vi "Configure Device.vi"(8 "error in":errorcluster, 11 "Alicat Device in":refnum<class "Alicat Device.lvclass">) -> (0 "error out":errorcluster, 3 "Alicat Device out":refnum<class "Alicat Device.lvclass">)   [LabVIEW 2015, in "Alicat Device.lvclass"]
uses:
  Alicat Device.lvclass
  Configurable Device/Configurable Device.lvclass/Configurable Device.ctl
  Reusable/Session APIs/File Access/Config Data/Config Data.lvclass/Config Data.ctl
  Alicat Device.lvclass/Alicat Device.ctl
  Configurable Device/Read Handle.vi
  <vilib>/Utility/config.llb/Read Key (String).vi
  <vilib>/Utility/config.llb/Read Key (Double).vi
  <vilib>/Utility/config.llb/Read Key (Boolean).vi
  Reusable/Session APIs/File Access/Config Data/Config Data.lvclass
  <vilib>/Utility/config.llb/NI_LVConfig.lvlib
  Reusable/Session APIs/Serial/Serial Session.lvclass
  <userlib>/_Session Fwk/Session - Root.lvclass
  Configurable Device/Configurable Device.lvclass
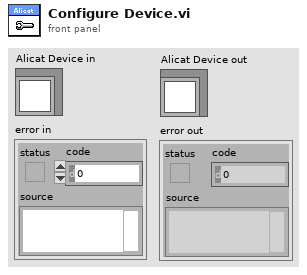
[diagram p1: front panel]
types:
  T1 = typedef "Config Data.lvclass/Config Session.ctl" = refnum<data-value>
  T2 = typedef "NI_LVConfig.lvlib/Config Data RefNum.ctl" = refnum<k1>
  T3 = typedef "Session - Root.lvclass/Session Handle.ctl" = refnum<data-value>
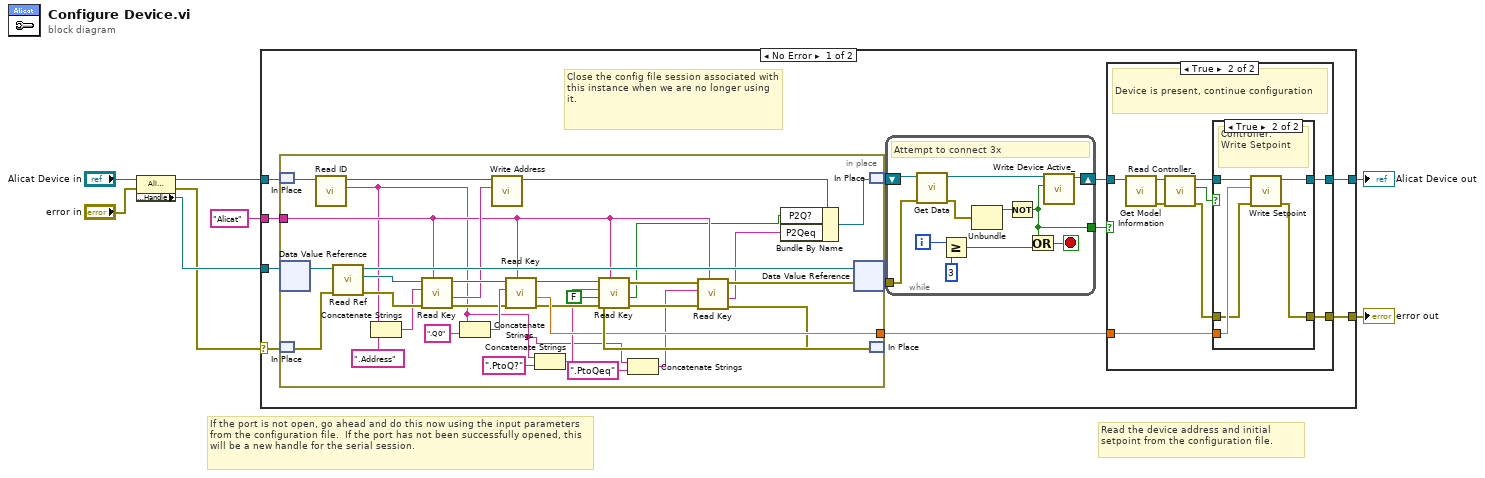
[diagram p0: block diagram]
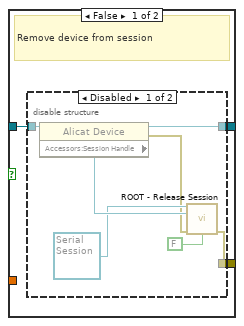
[diagram p2: hidden frame]
diagram:
  # "If the port is not open, go ahead and do this now using the input parameters from the configuration file.  If the port has not been successfully opened, this will be a new handle for the serial session."
  # "Read the device address and initial setpoint from the configuration file."
  n1 = property class="Alicat Device"(reference="Alicat Device in", error in="error in") -> (reference out=w5:refnum<class "Alicat Device.lvclass">, error out=w7:errorcluster, "Accessors:Handle"=w8:T1)
  n2 = case shown="No Error" w7 {
    selector: w7 -> [w12 w89]
    tunnel: w8 -> [w9 _]
    tunnel: "Alicat" ("section") -> [w19 _]
    tunnel: [w17 w89] -> w1
    tunnel: [w14 w90] -> w2
    tunnel: w5 -> [w13 w90]
    frame No Error {
      # "Close the config file session associated with this instance when we are no longer using it."
      n3 = in-place {
        in-place-border: w19 -> [w69]
        in-place-border: [w74] -> w15
        n4 = in-place-match #1(w13) -> (w77:refnum<class "Alicat Device.lvclass">)
        n5 = in-place-dvr #2(w9) -> (w88:refnum<class "Config Data.lvclass">)  [unwired: 1 out]
        n6 = in-place-match #3(w12) -> (w87:errorcluster)
        n7 = call "Read ID.vi"("Alicat Device in"=w77) -> ("ID"=w58:string, "Alicat Device out"=w76:refnum<class "Alicat Device.lvclass">)  [unwired: 8 in, 1 out]
        n8 = call "Read Ref.vi"("error in (no error)"=w87, "Config Data in"=w88) -> ("error out"=w85:errorcluster, "config data"=w86:T2, "Config Data out"=w78:refnum<class "Config Data.lvclass">)  [unwired: 7 in]
        n9 = Concatenate Strings(w58, ".Address" ("string")) -> (w83:string)
        n10 = call-poly <vilib>:"Read Key.vi"("section"=w69, "error in (no error)"=w85, "key"=w83, "refnum"=w86) -> ("error out"=w79:errorcluster, "value"=w75:string, "refnum out"=w82:T2)  [unwired: 4 in, 1 out]
        n11 = Concatenate Strings(w58, ".Q0" ("string")) -> (w80:string)
        n12 = call "Write Address.vi"("Address"=w75, "Alicat Device in"=w76) -> ("Alicat Device out"=w63:refnum<class "Alicat Device.lvclass">)  [unwired: 8 in, 1 out]
        n13 = call-poly <vilib>:"Read Key.vi"("section"=w69, "error in (no error)"=w79, "key"=w80, "refnum"=w82) -> ("error out"=w71:errorcluster, "value"=w74:dbl, "refnum out"=w73:T2)  [unwired: 4 in, 1 out]
        n14 = Concatenate Strings(w58, ".PtoQ?" ("string")) -> (w67:string)
        n15 = call-poly <vilib>:"Read Key.vi"("section"=w69, "error in (no error)"=w71, "default value"=FALSE, "key"=w67, "refnum"=w73) -> ("error out"=w70:errorcluster, "value"=w62:bool, "refnum out"=w72:T2)  [unwired: 3 in, 1 out]
        n16 = Concatenate Strings(w58, ".PtoQeq" ("string")) -> (w64:string)
        n17 = call-poly <vilib>:"Read Key.vi"("section"=w69, "error in (no error)"=w70, "key"=w64, "refnum"=w72) -> ("error out"=w60:errorcluster, "value"=w61:string)  [unwired: 4 in, 2 out]
        n18 = Bundle By Name(cluster=w63, "P2Q?"=w62, "P2Qeq"=w61) -> (w59:refnum<class "Alicat Device.lvclass">)
        n19 = in-place-dvr #2(w78) -> ()  [unwired: 2 out]
        n20 = in-place-match #1(w59) -> (w18:refnum<class "Alicat Device.lvclass">)
        n21 = in-place-match #3(w60) -> (w10:errorcluster)
      }
      n22 = while {
        shift-right: [w48] -> w16
        shift-left: w18 -> [w53]
        tunnel: [w47] -> w11
        tunnel: w10 -> [w50]
        i -> [w51]
        stop <- w54 stop-if-true
        # "Attempt to connect 3x"
        n23 = call-dynamic "Get Data.vi"("error in"=w50, "Cfg Dev in"=w53) -> ("error out"=w52:errorcluster, "Cfg Dev out"=w49:refnum<class "Alicat Device.lvclass">)  [unwired: 7 in, 1 out]
        n24 = Greater Or Equal?(x=w51, y=3) -> (x >= y?=w56:bool)
        n25 = Unbundle(w52) -> ("status"=w55:bool)  [unwired: 2 out]
        n26 = Not(x=w55) -> (.not. x?=w47:bool)
        n27 = Or(x=w47, y=w56) -> (x .or. y?=w54:bool)
        n28 = call "Write Device Active_.vi"("Device Active?"=w47, "Configurable Device in"=w49) -> ("Configurable Device out"=w48:refnum<class "Alicat Device.lvclass">)  [unwired: 8 in, 1 out]
      }
      n29 = case shown="True" w11 {
        tunnel: [w20 w32] -> w17
        tunnel: w16 -> [w22 w39]
        tunnel: w15 -> [_ w33]
        tunnel: [w21 w31] -> w14
        frame False {
          # "Remove device from session"
          n30 = disable-structure shown="Disabled" {
            disable-tunnel: w22 -> [w29 w30]
            disable-tunnel: [w28 w30] -> w21
            disable-tunnel: [w25 _] -> w20
            frame Disabled {
              n31 = property class="Alicat Device"(reference=w29) -> (reference out=w28:refnum<class "Alicat Device.lvclass">, error out=w24:errorcluster, "Accessors:Session Handle"=w27:T3)  [unwired: 1 in]
              n32 = call <userlib>:"ROOT - Release Session.vi"("OBJ - Session in"=refnum<class "Serial Session.lvclass"> refnum ("Serial Session in"), "Session Handle in"=w27, "error in (no error)"=w24, "force destroy? (F)"=FALSE) -> ("error out"=w25:errorcluster)  [unwired: 10 in, 1 out]
            }
            frame Enabled {
            }
          }
        }
        frame True {
          # "Device is present, continue configuration"
          n33 = call "Get Model Information.vi"("Alicat Device in"=w39) -> ("error out"=w37:errorcluster, "Alicat Device out"=w38:refnum<class "Alicat Device.lvclass">)  [unwired: 8 in, 1 out]
          n34 = call "Read Controller_.vi"("error in"=w37, "Alicat Device in"=w38) -> ("error out"=w35:errorcluster, "Controller?"=w36:bool, "Alicat Device out"=w34:refnum<class "Alicat Device.lvclass">)  [unwired: 7 in]
          n35 = case shown="True" w36 {
            tunnel: w35 -> [w40 w44]
            tunnel: w34 -> [w41 w46]
            tunnel: w33 -> [_ w45]
            tunnel: [w40 w43] -> w32
            tunnel: [w41 w42] -> w31
            frame False {
            }
            frame True {
              # "Controller:\nWrite Setpoint"
              n36 = call "Write Setpoint.vi"("error in"=w44, "Setpoint"=w45, "Alicat Device in"=w46) -> ("error out"=w43:errorcluster, "Alicat Device out"=w42:refnum<class "Alicat Device.lvclass">)  [unwired: 6 in, 1 out]
            }
          }
        }
      }
    }
    frame Error {
    }
  }
  "error out" <- w1
  "Alicat Device out" <- w2
